vi "Refresh Aux Listbox.vi"(4 "Serial Aux In 9-16":T1, 6 "Serial Aux In 1-8":T1, 8 "Filters":sgl[](array[numeric]), 9 "Names":string[](array[string]), 11 "MulticolumnListbox in":refnum<vi>) -> ()   [LabVIEW 2016, in "DCM System Explorer.lvlib"]
uses:
  DCM System Explorer.lvlib
  <vilib>/Powertrain Controls/Device Drivers/DCM/Rev0/FPGA/Digital Channel.ctl
  <vilib>/Powertrain Controls/Device Drivers/DCM/Rev0/FPGA/DCM - FPGA.lvlib
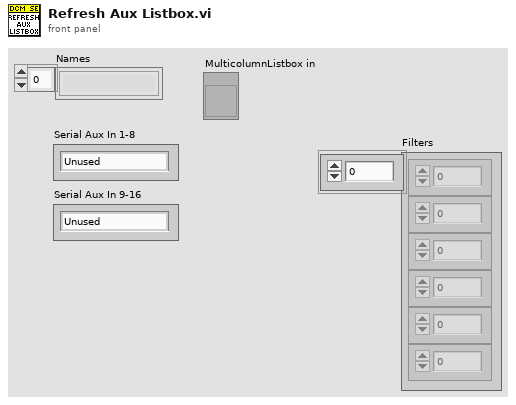
[diagram p1: front panel]
types:
  T1 = typedef "DCM - FPGA.lvlib/Digital Channel.ctl" = enum8{"Unused", "User OS", "Diff IO 1", "Diff IO 2", "Diff IO 3", "Diff IO 4", "Diff IO 5", "Diff IO 6", "Diff IO 7", "Diff IO 8", "Aux 1", "Aux 2", "Aux 3", "Aux 4", "Aux 5", "Aux 6", "Aux 7", "Aux 8", "Aux 9", "Aux 10", "Aux 11", "Aux 12", "Aux 13", "Aux 14", "Aux 15", "Aux 16"}
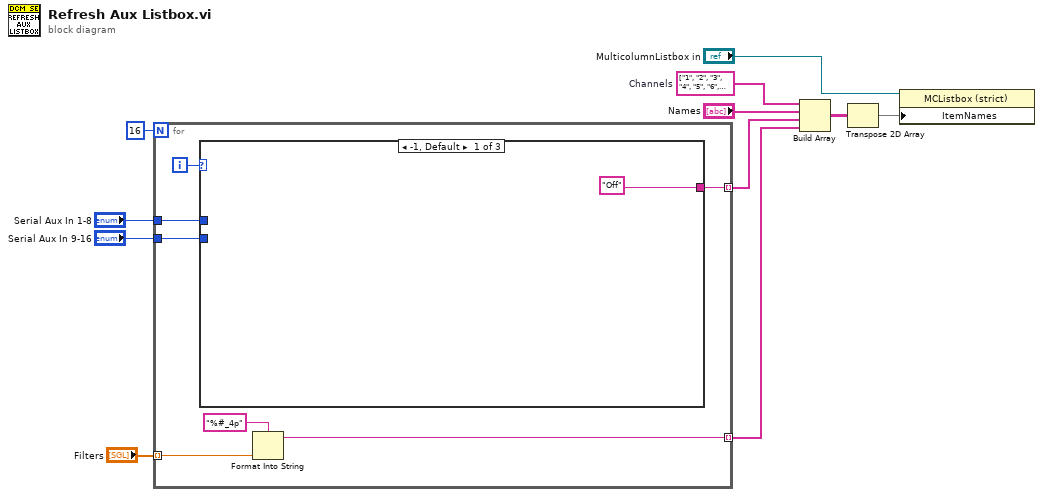
[diagram p0: block diagram]
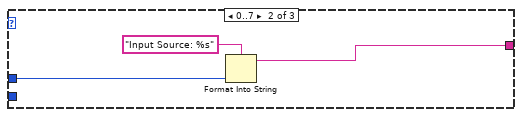
[diagram p2: hidden frame]
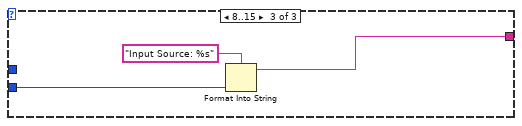
[diagram p3: hidden frame]
diagram:
  w10 = string[] ["1", "2", "3", "4", "5", "6", "7", "8", "9", "10", "11", "12", "13", "14", "15", "16"]  # Channels
  n1 = for {
    N: 16 -> [_]
    tunnel: [w16] -> w5 mode=indexing
    tunnel: "Filters" -> [w18] mode=indexing
    tunnel: [w17] -> w4 mode=indexing
    tunnel: "Serial Aux In 1-8" -> [w13]
    tunnel: "Serial Aux In 9-16" -> [w14]
    i -> [w15]
    n2 = case shown="-1, Default" w15 {
      tunnel: ["Off" ("format string") w20 w24] -> w16
      tunnel: w13 -> [_ w22 _]
      tunnel: w14 -> [_ _ w23]
      frame -1, Default {
      }
      frame 0..7 {
        n3 = Format Into String(format string="Input Source: %s", w22) -> (resulting string=w20:string)  [unwired: 2 in, 1 out]
      }
      frame 8..15 {
        n4 = Format Into String(format string="Input Source: %s", w23) -> (resulting string=w24:string)  [unwired: 2 in, 1 out]
      }
    }
    n5 = Format Into String(format string="%#_4p", w18) -> (resulting string=w17:string)  [unwired: 2 in, 1 out]
  }
  n6 = Build Array(w10, "Names", w5, w4) -> (w11:string[][])
  n7 = Transpose 2D Array(2D array=w11) -> (transposed array=w9:string[][])
  n8 = property on="Property Node" class="MCListbox (strict)"(reference="MulticolumnListbox in", "ItemNames"=w9) -> ()  [unwired: 1 in, 2 out]
